vi "ExXCamerasSameGraph.vi"() -> ()   [LabVIEW 2010]
panel:
  in  "Number of Cameras":u32=1 min=1 max=20 step=1
  out "Camera 16":sgl[](graph)
  out "Camera 15":sgl[](graph)
  out "Camera 14":sgl[](graph)
  out "Camera 13":sgl[](graph)
  out "Camera 12":sgl[](graph)
  out "Camera 11":sgl[](graph)
  out "Camera 10":sgl[](graph)
  out "Camera 9":sgl[](graph)
  out "Camera 8":sgl[](graph)
  out "Camera 7":sgl[](graph)
  out "Camera 6":sgl[](graph)
  out "Camera 5":sgl[](graph)
  out "Camera 4":sgl[](graph)
  out "Camera 3":sgl[](graph)
  out "Camera 2":sgl[](graph)
  out "Camera 1":sgl[](graph)
  in  "stop":bool
  in  "Exposure":dbl=0.5 format="%.2f"
  out "error out":errorcluster
  in  "error in (no error)":errorcluster
  # "Ex2CamerasSameGraph:\nThis example runs two cameras in focus mode.\nSets them up for center strip and displays as graph.\nRemember to setup two cameras in the pvcam.ini\nfile."
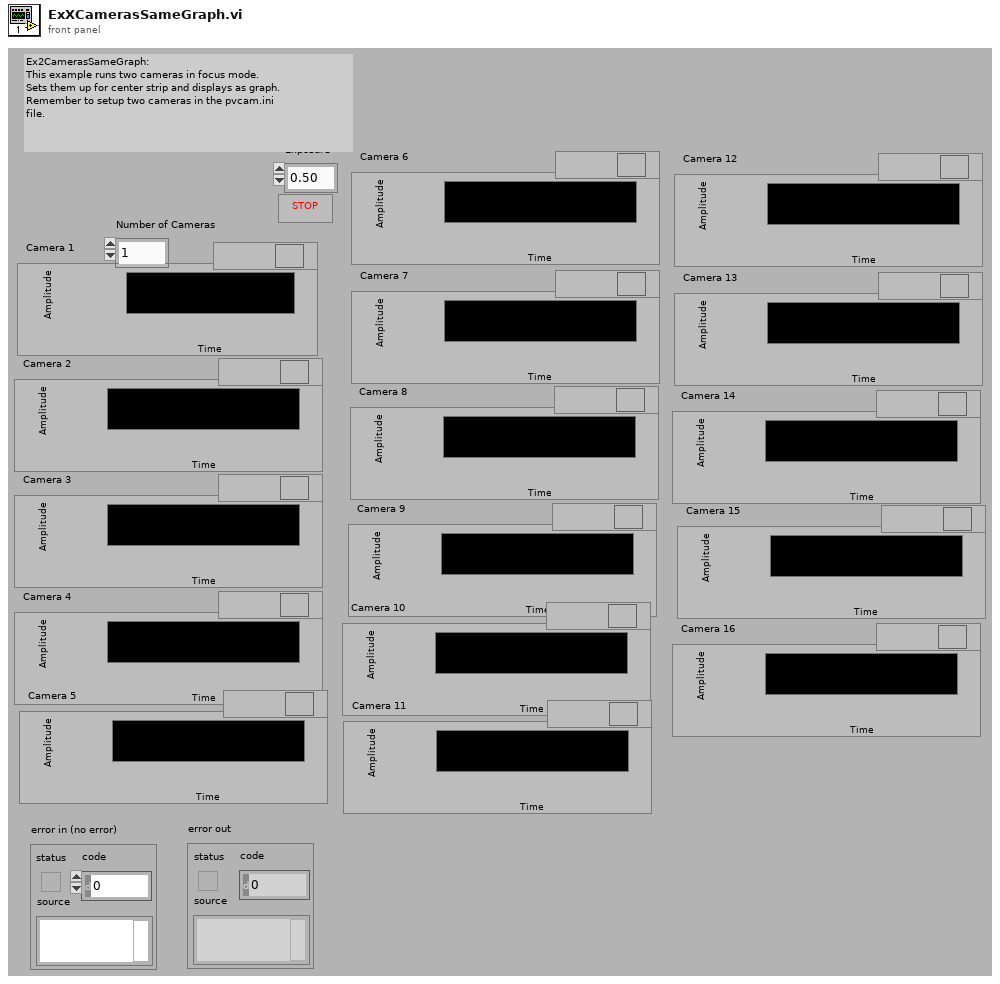
[diagram p1: front panel]
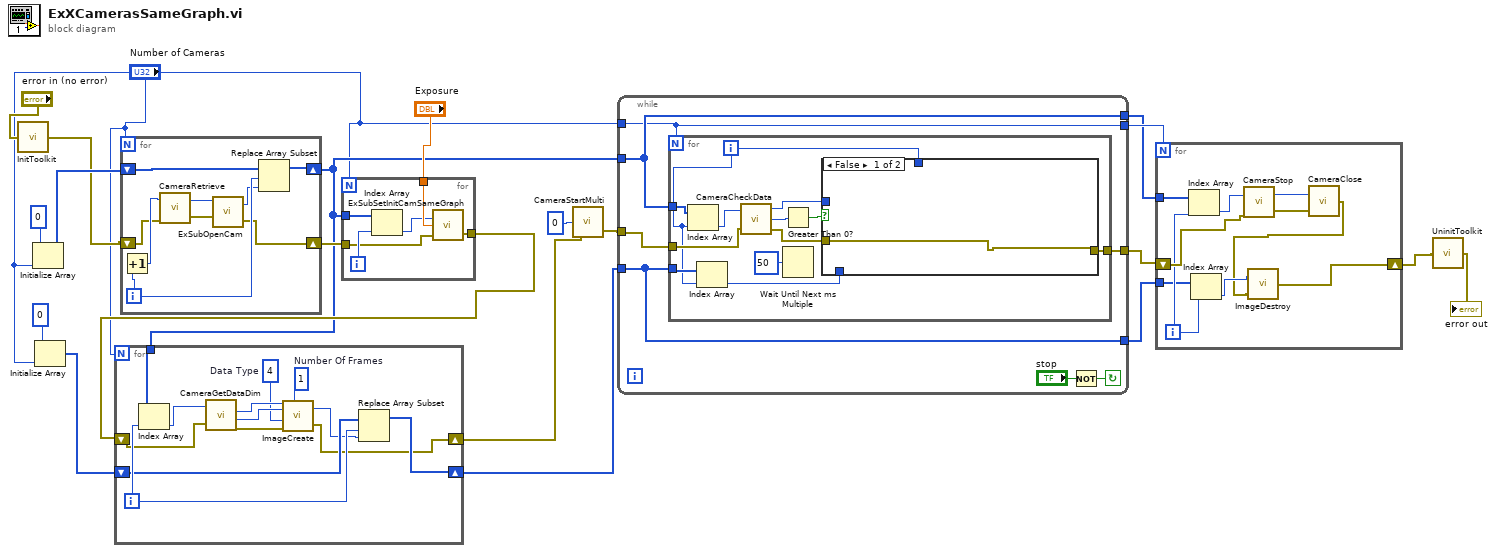
[diagram p0: block diagram]
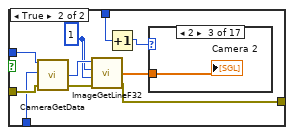
[diagram p2: hidden frame]
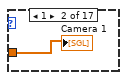
[diagram p4: hidden frame]
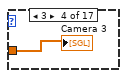
[diagram p5: hidden frame]
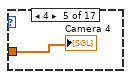
[diagram p6: hidden frame]
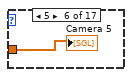
[diagram p7: hidden frame]
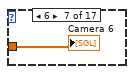
[diagram p8: hidden frame]
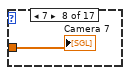
[diagram p9: hidden frame]
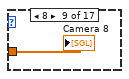
[diagram p10: hidden frame]
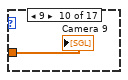
[diagram p11: hidden frame]
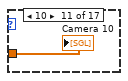
[diagram p12: hidden frame]
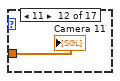
[diagram p13: hidden frame]
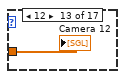
[diagram p14: hidden frame]
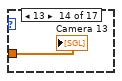
[diagram p15: hidden frame]
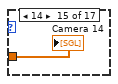
[diagram p16: hidden frame]
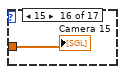
[diagram p17: hidden frame]
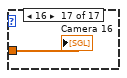
[diagram p18: hidden frame]
diagram:
  n1 = call <userlib>:"InitToolkit.vi"("error in"="error in (no error)") -> ("error out"=w13:errorcluster)
  n2 = Initialize Array(0, "Number of Cameras") -> (w15:i32[])
  n3 = Initialize Array(0, "Number of Cameras") -> (w11:i32[])
  n4 = for {
    N: "Number of Cameras" -> [_]
    shift-right: [w25] -> w6
    shift-left: w15 -> [w27]
    shift-right: [w22] -> w14
    shift-left: w13 -> [w28]
    i -> [w30]
    n5 = Increment(x=w30) -> (x+1=w29:i32)
    n6 = call <userlib>:"CameraRetrieve.vi"("error in"=w28, "Camera Index"=w29) -> ("error out"=w23:errorcluster, "Device ID"=w26:u32)
    n7 = call "ExSubOpenCam.vi"("error in (no error)"=w23, "Camera Device ID"=w26) -> ("error out"=w22:errorcluster, "Camera Handle"=w24:u32)
    n8 = Replace Array Subset(array=w27, new element=w24, index=w30) -> (w25:i32[])
  }
  n9 = for {
    N: "Number of Cameras" -> [_]
    tunnel: w6 -> [w36]
    tunnel: w14 -> [w32]
    tunnel: [w34] -> w10
    tunnel: "Exposure" -> [w33]
    i -> [w35]
    n10 = Index Array(array=w36, index=w35) -> (element=w31:i32)
    n11 = call "ExSubSetInitCamSameGraph.vi"("error in (no error)"=w32, "Exposure"=w33, "Camera Handle"=w31) -> ("error out"=w34:errorcluster)  [unwired: 1 out]
  }
  n12 = for {
    N: "Number of Cameras" -> [_]
    shift-right: [w38] -> w7
    shift-left: w11 -> [w40]
    shift-right: [w37] -> w9
    shift-left: w10 -> [w46]
    tunnel: w6 -> [w49]
    i -> [w48]
    w44 = u32 1  # Number Of Frames
    w41 = u32 4  # Data Type
    n13 = Index Array(array=w49, index=w48) -> (element=w47:i32)
    n14 = call <userlib>:"CameraGetDataDim.vi"("Camera Handle"=w47, "error in"=w46) -> ("Xdim"=w43:u32, "Ydim"=w42:u32, "error out"=w45:errorcluster)  [unwired: 1 out]
    n15 = call <userlib>:"ImageCreate.vi"("X dimension"=w43, "Y dimension"=w42, "Data Type"=w41, "error in"=w45, "Number Of Frames"=w44) -> ("Image Handle"=w39:u32, "error out"=w37:errorcluster)
    n16 = Replace Array Subset(array=w40, new element=w39, index=w48) -> (w38:i32[])
  }
  n17 = call "CameraStartMulti.vi"("error in (no error)"=w9, "Number Of Cameras"=0) -> ("error out"=w19:errorcluster)  [unwired: 1 in, 1 out]
  n18 = while {
    tunnel: w19 -> [w54]
    tunnel: w6 -> [w52]
    tunnel: [w53] -> w1
    tunnel: "Number of Cameras" -> [w50]
    tunnel: w7 -> [w51]
    tunnel: [w52] -> w3
    tunnel: [w51] -> w2
    tunnel: [w50] -> w4
    stop <- w55 continue-if-true
    n19 = for {
      N: w50 -> [_]
      tunnel: [w63] -> w53
      tunnel: w52 -> [w62]
      tunnel: w54 -> [w60]
      tunnel: w51 -> [w59]
      i -> [w57]
      n20 = Index Array(array=w62, index=w57) -> (element=w61:i32)
      n21 = Index Array(array=w59, index=w57) -> (element=w58:i32)
      n22 = call <userlib>:"CameraCheckData.vi"("Camera Handle"=w61, "error in"=w60) -> ("Camera Handle"=w65:u32, "Number Of Frames Available"=w67:i32, "error out"=w64:errorcluster)
      n23 = Greater Than 0?(x=w67) -> (x > 0?=w66:bool)
      n24 = Wait Until Next ms Multiple(millisecond multiple=u32 50) -> ()  [unwired: 1 out]
      n25 = case shown="False" w66 {
        tunnel: [w69 w76] -> w63
        tunnel: w65 -> [_ w75]
        tunnel: w64 -> [w69 w74]
        tunnel: w57 -> [_ w70]
        tunnel: w58 -> [_ w72]
        frame False {
        }
        frame True {
          w77 = 1
          n26 = call <userlib>:"CameraGetData.vi"("error in"=w74, "Data Handle"=w72, "Camera Handle"=w75) -> ("error out"=w79:errorcluster, "Data Handle"=w78:u32)  [unwired: 1 out]
          n27 = call <userlib>:"ImageGetLineF32.vi"("error in"=w79, "Z Position"=w77, "Y Position"=w77, "Data Handle"=w78) -> ("error out"=w76:errorcluster, "Array F32"=w73:sgl[])  [unwired: 1 out]
          n28 = Increment(x=w70) -> (x+1=w71:i32)
          n29 = case shown="2" w71 {
            tunnel: w73 -> [_ w80 w81 w82 w83 w84 w85 w86 w87 w88 w89 w90 w91 w92 w93 w94 w95]
            frame Default {
            }
            frame 1 {
              "Camera 1" <- w80
            }
            frame 2 {
              "Camera 2" <- w81
            }
            frame 3 {
              "Camera 3" <- w82
            }
            frame 4 {
              "Camera 4" <- w83
            }
            frame 5 {
              "Camera 5" <- w84
            }
            frame 6 {
              "Camera 6" <- w85
            }
            frame 7 {
              "Camera 7" <- w86
            }
            frame 8 {
              "Camera 8" <- w87
            }
            frame 9 {
              "Camera 9" <- w88
            }
            frame 10 {
              "Camera 10" <- w89
            }
            frame 11 {
              "Camera 11" <- w90
            }
            frame 12 {
              "Camera 12" <- w91
            }
            frame 13 {
              "Camera 13" <- w92
            }
            frame 14 {
              "Camera 14" <- w93
            }
            frame 15 {
              "Camera 15" <- w94
            }
            frame 16 {
              "Camera 16" <- w95
            }
          }
        }
      }
    }
    n30 = Not(x="stop") -> (.not. x?=w55:bool)
  }
  n31 = for {
    N: w4 -> [_]
    shift-right: [w105] -> w8
    shift-left: w1 -> [w104]
    tunnel: w3 -> [w102]
    tunnel: w2 -> [w101]
    i -> [w103]
    n32 = Index Array(array=w102, index=w103) -> (element=w99:i32)
    n33 = Index Array(array=w101, index=w103) -> (element=w100:i32)
    n34 = call <userlib>:"CameraStop.vi"("error in"=w104, "Camera Handle"=w99) -> ("error out"=w98:errorcluster, "Camera Handle"=w96:u32)
    n35 = call <userlib>:"CameraClose.vi"("error in"=w98, "Camera Handle"=w96) -> ("error out"=w97:errorcluster)
    n36 = call <userlib>:"ImageDestroy.vi"("error in"=w97, "Data handle"=w100) -> ("error out"=w105:errorcluster)
  }
  n37 = call <userlib>:"UninitToolkit.vi"("error in"=w8) -> ("error out"=→"error out":errorcluster)
